vi "Hardware-acquisition-loop.vi"(4 "Timeout":timestamp, 6 "Acquisition notif":refnum<notifier>, 8 "error in (no error)":errorcluster, 9 "Buffers":refnum<class "CV-Buffers.lvclass">, 10 "Config. params. ref. in":refnum<data-value>, 11 "Acquis. params. ref. in":refnum<data-value>) -> (0 "error out":errorcluster, 2 "Config. params. ref.":refnum<data-value>, 3 "Acquis. params. ref.":refnum<data-value>)   [LabVIEW 2013, in "CameraVision.lvlib" / "CV-Acquisition.lvclass"]
uses:
  CV-Acquisition.lvclass
  Configuration/CV-Configuration.lvclass
  Buffers/CV-Buffers.lvclass
  <vilib>/Platform/TimedLoop/XDataNode/timing_clust.ctl
  <vilib>/Platform/TimedLoop/XDataNode/nitl_modes.ctl
  <vilib>/Platform/TimedLoop/XDataNode/wakeup.ctl
  <vilib>/Platform/TimedLoop/XDataNode/XDataNode.xnode
  <vilib>/Platform/TimedLoop/XDataNode/XDNodeRunTimeDep.lvlib
  CV-Main.lvclass
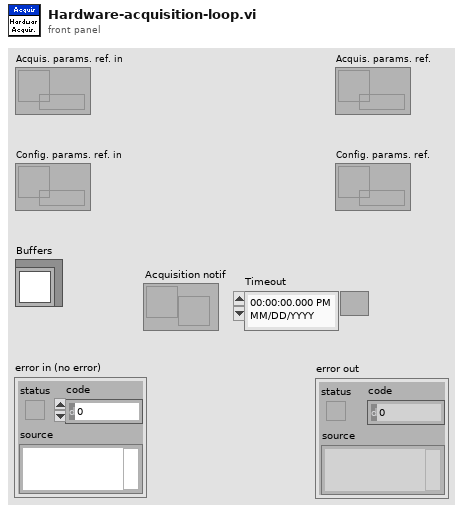
[diagram p1: front panel]
types:
  T1 = typedef "XDNodeRunTimeDep.lvlib/timing_clust.ctl" = cluster{"Expected End [f-1]":u64, "Actual End [f-1]":u64, "Finished Late? [f-1]":bool, "Expected End [i-1]":u64, "Actual End [i-1]":u64, "Finished Late? [i-1]":bool, "Expected Start [i]":u64, "Actual Start [i]":u64, "Expected Start [f]":u64, "Actual Start [f]":u64, "Source Name":string, "Structure Name":string, "Period":i64, "Deadline":i64, "Offset":i64, "Start":i64, "Priority":i32, "Timeout":i32, "Mode":T2, "Wakeup Reason":T3, "Error":errorcluster, "Source Type":string, "Secondary Source Type":string, "Global End Time":u64, "Global Start Time":u64, "Frame Duration":u64, "Iteration Duration":u64, "Assigned CPU":i32, "I/O Scan Engine Mode":u32}
  T2 = typedef "XDNodeRunTimeDep.lvlib/nitl_modes.ctl" = enum32{"No Change", "Process missed periods, maintain original phase", "Discard missed periods, maintain original phase", "Process missed periods, ignore original phase", "Discard missed periods, ignore original phase"}
  T3 = typedef "XDNodeRunTimeDep.lvlib/wakeup.ctl" = enum32{"Normal", "Aborted", "Asynchronous wakeup", "Timing source error", "Timed loop error", "Timeout"}
  T4 = typedef "IMAQ Image.ctl" = refnum<image>
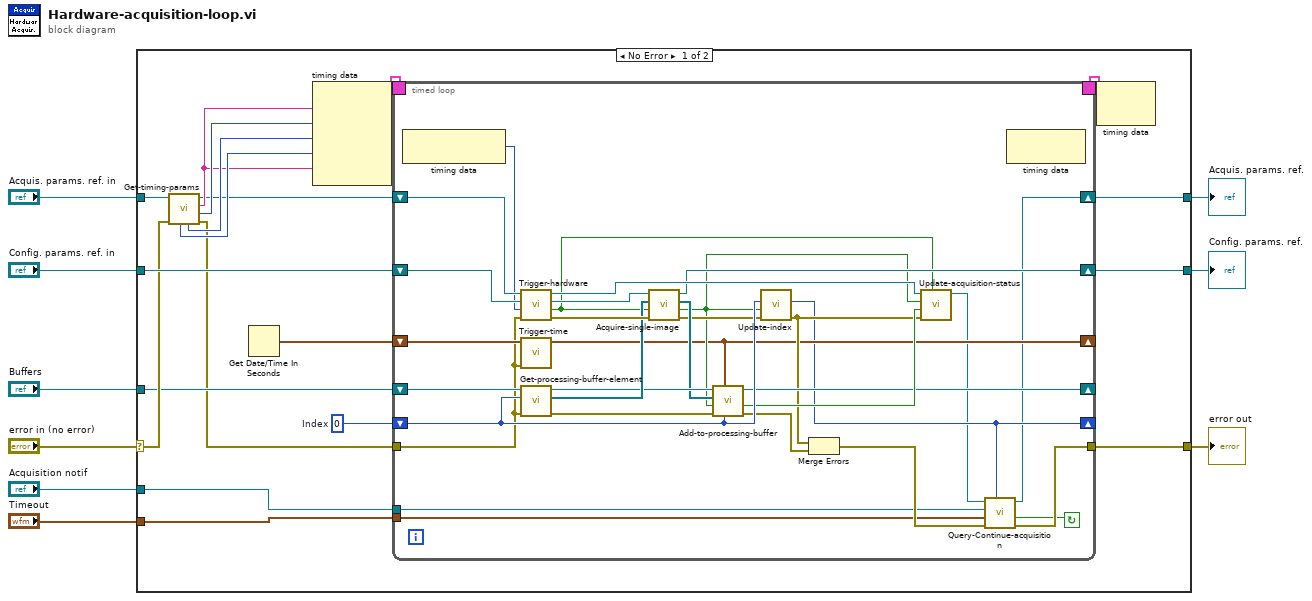
[diagram p0: block diagram]
diagram:
  n1 = case shown="No Error" "error in (no error)" {
    selector: "error in (no error)" -> [w21 w73]
    tunnel: [w18 w73] -> w8
    tunnel: "Acquis. params. ref. in" -> [w24 w72]
    tunnel: [w19 w71] -> w4
    tunnel: [w20 w72] -> w6
    tunnel: "Config. params. ref. in" -> [w22 w71]
    tunnel: "Buffers" -> [w14 _]
    tunnel: "Acquisition notif" -> [w12 _]
    tunnel: "Timeout" -> [w11 _]
    frame No Error {
      w17 = 0  # Index
      n2 = call "Get-timing-params.vi"("error in (no error)"=w21, "Acquis. params. ref. in"=w24) -> ("error out"=w13:errorcluster, "Period"=w26:i64, "Source"=w15:string, "Acquis. params. ref."=w10:refnum<data-value>, "Timeout"=w25:i32, "Mode"=w23:T2)  [unwired: 4 in]
      n3 = Get Date/Time In Seconds() -> (seconds since 1Jan1904=w16:timestamp)
      n4 = node-c288(w15, w26, w25, w23, w15) -> (w28:T1)
      n5 = timed-loop {
        timing: w28 -> [_]
        timing-out: [_] -> w27
        shift-right: [w29] -> w20
        shift-left: w10 -> [w59]
        shift-right: [w46] -> w19
        shift-left: w22 -> [w58]
        shift-right: [w32] -> _
        shift-left: w17 -> [w50]
        shift-right: [w47] -> _
        shift-left: w14 -> [w56]
        tunnel: w13 -> [w35]
        tunnel: [w43] -> w18
        shift-right: [w34] -> _
        shift-left: w16 -> [w36]
        tunnel: w12 -> [w30]
        tunnel: w11 -> [w33]
        stop <- w42 continue-if-true
        n6 = node-c288() -> (w57:T3)  [unwired: 1 in]
        n7 = call "Trigger-hardware.vi"("error in (no error)"=w35, "Wakeup Reason"=w57, "Config. params. ref. in"=w58, "Acquis. params. ref. in"=w59) -> ("error out"=w54:errorcluster, "Tigger ok?"=w38:bool, "Config. params. ref."=w55:refnum<data-value>, "Acquis. params. ref."=w49:refnum<data-value>)  [unwired: 4 in]
        n8 = call "Trigger-time.vi"("error in (no error)"=w35, "Previous time"=w36) -> ("Trigger time"=w34:timestamp)  [unwired: 9 in]
        n9 = call "Get-processing-buffer-element.vi"("error in (no error)"=w35, "Index"=w50, "Buffers in"=w56) -> ("error out"=w51:errorcluster, "Element ref"=w53:T4[], "Buffers out"=w52:refnum<class "CV-Buffers.lvclass">)  [unwired: 6 in]
        n10 = call "Acquire-single-image.vi"("error in (no error)"=w54, "Trigger ok?"=w38, "Images in"=w53, "Config. params. ref. in"=w55) -> ("error out"=w40:errorcluster, "Image ok?"=w37:bool, "Images"=w41:T4[], "Config. params. ref."=w46:refnum<data-value>)  [unwired: 4 in]
        n11 = call "Add-to-processing-buffer.vi"("Index"=w50, "Time"=w34, "error in (no error)"=w51, "Image ok?"=w37, "Images"=w41, "Buffers in"=w52) -> ("error out"=w39:errorcluster, "Buffer ok?"=w48:bool, "Buffers out"=w47:refnum<class "CV-Buffers.lvclass">)  [unwired: 3 in]
        n12 = call "Update-index.vi"("error in (no error)"=w40, "Image ok?"=w37, "Index in"=w50) -> ("error out"=w45:errorcluster, "Index"=w32:i32)  [unwired: 7 in]
        n13 = Merge Errors(w45, w39) -> (w44:errorcluster)
        n14 = call "Update-acquisition-status.vi"("Tigger ok?"=w38, "error in (no error)"=w45, "Queue ok?"=w48, "Image ok?"=w37, "Acquis. params. ref. in"=w49) -> ("Acquis. params. ref."=w31:refnum<data-value>)  [unwired: 5 in, 1 out]
        n15 = call "Query-Continue-acquisition.vi"("Index"=w32, "error in"=w44, "Timeout"=w33, "Acquisition notif"=w30, "Acquis. params. ref. in"=w31) -> ("error IO"=w43:errorcluster, "Continue?"=w42:bool, "Acquis. params. ref."=w29:refnum<data-value>)  [unwired: 4 in]
        n16 = node-c288() -> ()  [unwired: 1 in, 1 out]
      }
      n17 = node-c288(w27) -> ()  [unwired: 1 out]
    }
    frame Error {
    }
  }
  "error out" <- w8
  "Acquis. params. ref." <- w6
  "Config. params. ref." <- w4
